vi "Configure OSC CURRent OFFSet query.vi"(8 "error in (no error)":errorcluster, 9 "Current range":u16=1 min=1 max=3 step=1, 10 "Step":u16=1 min=1 max=99 step=1, 11 "VISA resource in":refnum<visa-resource-name>) -> (0 "error out":errorcluster, 2 "Offsert value":string, 3 "VISA resource out":refnum<visa-resource-name>)   [LabVIEW 2025, in "Chroma 19052.lvlib"]
doc: "This VI set the OPEN limit for Open/Short Circuit (OSC) test mode.\nRange: 0.1 to 1, step 0.1"
uses:
  <instrlib>/Chroma 19052/Chroma 19052.lvlib
panel:
  # "[F]"
  # "Query CURRENT OFFSET"
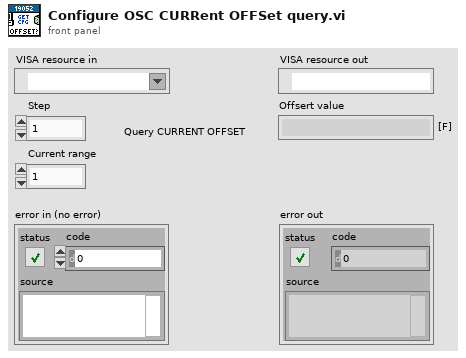
[diagram p1: front panel]
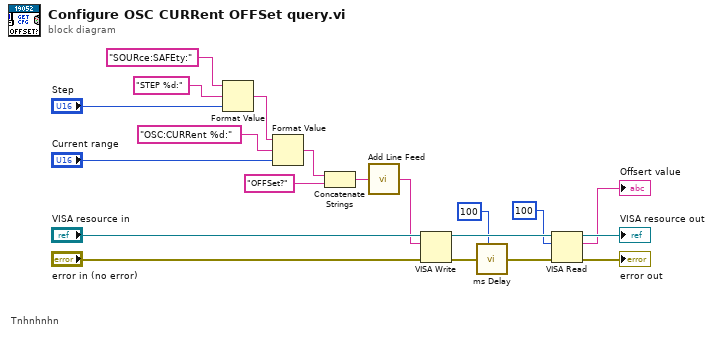
[diagram p0: block diagram]
diagram:
  # "Tnhnhnhn"
  n1 = Format Value(string ("")="SOURce:SAFEty:", format string="STEP %d:", value (0)="Step") -> (output string=w10:string)
  n2 = Format Value(string ("")=w10, format string="OSC:CURRent %d:", value (0)="Current range") -> (output string=w8:string)
  n3 = Concatenate Strings(w8, "OFFSet?" ("format string")) -> (w2:string)
  n4 = call <instrlib>:"Add Line Feed.vi"("Command string"=w2) -> ("Concatenated string"=w1:string)  [unwired: 4 in]
  n5 = VISA Write(VISA resource name="VISA resource in", write buffer=w1, error in (no error)="error in (no error)") -> (VISA resource name out=w7:refnum<visa-resource-name>, error out=w5:errorcluster)  [unwired: 1 out]
  n6 = call <instrlib>:"ms Delay.vi"("miliseconds to wait"=u32 100, "error in (no error)"=w5) -> ("error out"=w4:errorcluster)  [unwired: 6 in, 1 out]
  n7 = VISA Read(VISA resource name=w7, byte count=u32 100, error in (no error)=w4) -> (VISA resource name out=→"VISA resource out":refnum<visa-resource-name>, read buffer=→"Offsert value":string, error out=→"error out":errorcluster)  [unwired: 1 out]
